vi "Save BD Image.vi"(8 "Error In":errorcluster, 10 "Target BD Image Path":path, 11 "VI Path":path) -> (0 "Error Out":errorcluster)   [LabVIEW 2020, in "LMH-Toolbox.lvlib" / "LMH-Documentation.lvlib"]
uses:
  LMH-Documentation.lvlib
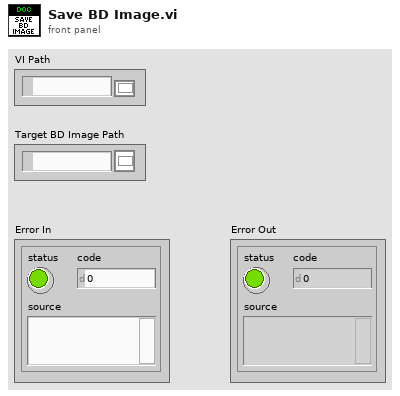
[diagram p1: front panel]
types:
  T1 = typedef "imagedata.ctl" = cluster{"image type":i32, "image depth":i32, "image":u8[], "mask":u8[], "colors":u32[], "Rectangle":cluster{"left":i16, "top":i16, "right":i16, "bottom":i16}}
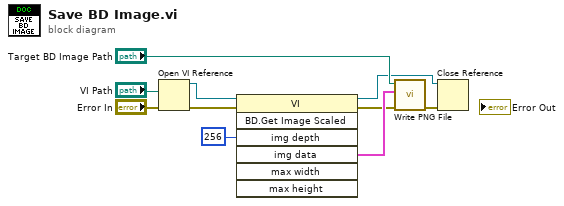
[diagram p0: block diagram]
diagram:
  n1 = Open VI Reference(vi path="VI Path", error in (no error)="Error In") -> (vi reference=w9:refnum<vi>, error out=w8:errorcluster)  [unwired: 4 in]
  n2 = invoke class="VI" method="BD.Get Image Scaled"(reference=w9, error in=w8, "img depth"=256 ("Image Depth")) -> (reference out=w2:refnum<vi>, error out=w4:errorcluster, "img data"=w6:T1)  [unwired: 4 in, 4 out]
  n3 = call <vilib>:"Write PNG File.vi"("error in (no error)"=w4, "image data"=w6, "path to PNG file"="Target BD Image Path") -> ("error out"=w3:errorcluster)  [unwired: 7 in, 1 out]
  n4 = Close Reference(reference=w2, error in (no error)=w3) -> ()  [unwired: 1 out]
